vi "GET_CALIB.vi"(0 "VISA resource name":refnum<visa-resource-name>, 1 "Gain":i8=1 min=1 max=3, 2 "error in (no error)":errorcluster) -> (3 "VISA resource Salida":refnum<visa-resource-name>, 4 "slope":dbl, 5 "offset":dbl, 6 "error out":errorcluster)   [LabVIEW 2011]
panel:
  out "unsigned byte array":u8[](array[numeric])
  out "leer comando get_Capture":u8[](array[numeric])
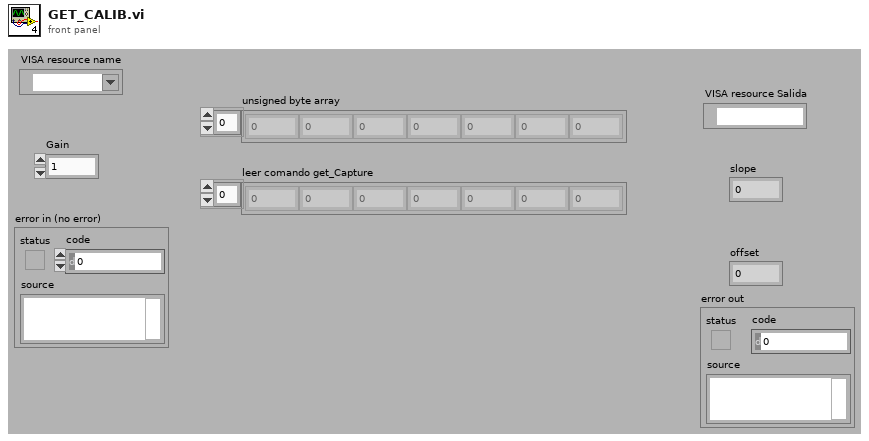
[diagram p1: front panel]
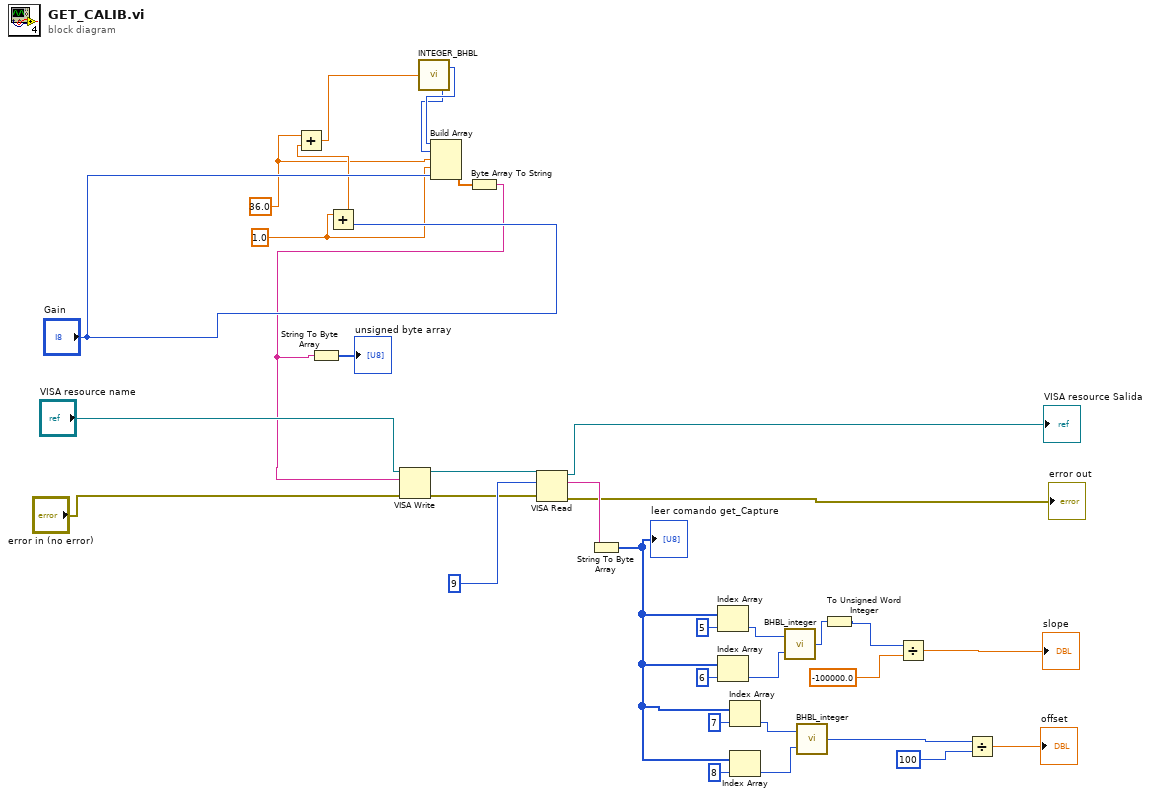
[diagram p0: block diagram]
diagram:
  w20 = 1.0 ("element")
  w18 = 36.0 ("element")
  n1 = Add(x=w20, y="Gain") -> (x+y=w19:dbl)
  n2 = Add(x=w18, y=w19) -> (x+y=w17:dbl)
  n3 = call "INTEGER_BHBL.vi"("int16"=w17) -> ("Lvalue"=w15:u8, "HValue"=w16:u8)
  n4 = Build Array(w16, w15, w18, w20, "Gain") -> (w28:dbl[])
  n5 = Byte Array To String(unsigned byte array=w28) -> (string=w14:string)
  n6 = String To Byte Array(string=w14) -> (unsigned byte array=→"unsigned byte array":u8[])
  n7 = VISA Write(VISA resource name="VISA resource name", write buffer=w14, error in (no error)="error in (no error)") -> (VISA resource name out=w29:refnum<visa-resource-name>, error out=w31:errorcluster)  [unwired: 1 out]
  n8 = VISA Read(VISA resource name=w29, byte count=u32 9, error in (no error)=w31) -> (VISA resource name out=→"VISA resource Salida":refnum<visa-resource-name>, read buffer=w33:string, error out=→"error out":errorcluster)  [unwired: 1 out]
  n9 = String To Byte Array(string=w33) -> (unsigned byte array=w8:u8[])
  "leer comando get_Capture" <- w8
  n10 = Index Array(array=w8, index=5) -> (element=w25:u8)
  n11 = Index Array(array=w8, index=6) -> (element=w24:u8)
  n12 = Index Array(array=w8, index=7) -> (element=w10:u8)
  n13 = Index Array(array=w8, index=8) -> (element=w9:u8)
  n14 = call "BHBL_integer.vi"("lo(x)"=w24, "hi(x)"=w25) -> ("(hi.lo)"=w2:i16)
  n15 = call "BHBL_integer.vi"("lo(x)"=w9, "hi(x)"=w10) -> ("(hi.lo)"=w5:i16)
  n16 = To Unsigned Word Integer(number=w2) -> (unsigned 16bit integer=w1:u16)
  n17 = Divide(x=w1, y=-100000.0) -> (x/y=→"slope":dbl)
  n18 = Divide(x=w5, y=i16 100) -> (x/y=→"offset":dbl)
